vi "throw.vi"(8 "exception in":T1 {"code" format="%.0x"}, 11 "code":i32) -> (0 "exception":T1 {"code" format="%.0x"})   [LabVIEW 2013, in "exception.lvlib"]
uses:
  exception.lvlib
  exception.ctl
  context.ctl
  const exceptioncausename.vi
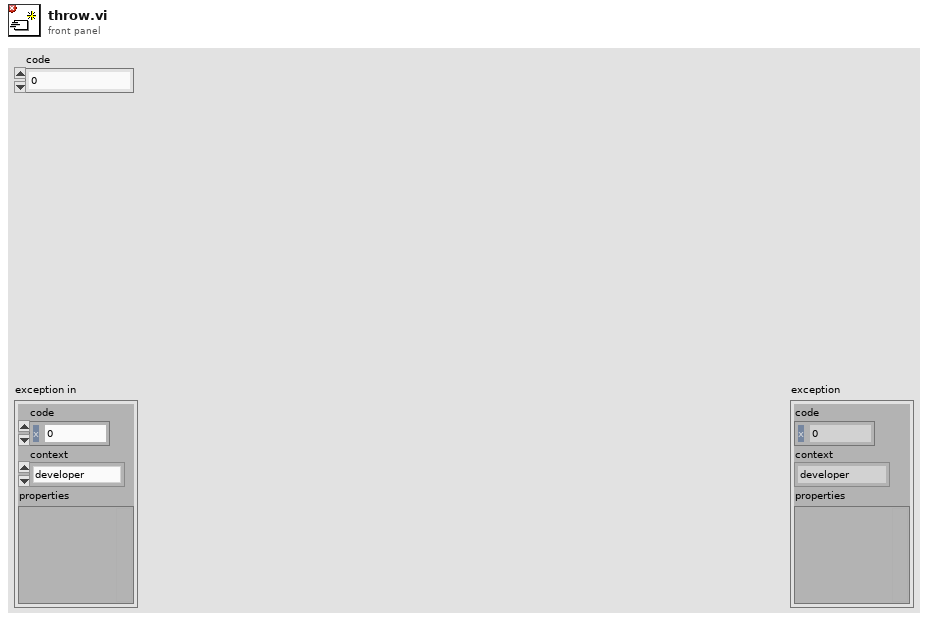
[diagram p1: front panel]
types:
  T1 = typedef "exception.lvlib/exception.ctl" = cluster{"code":i32, "context":T2, "properties":variant}
  T2 = typedef "exception.lvlib/context.ctl" = enum16{"developer", "user interface", "standard", "limited", "deterministic"}
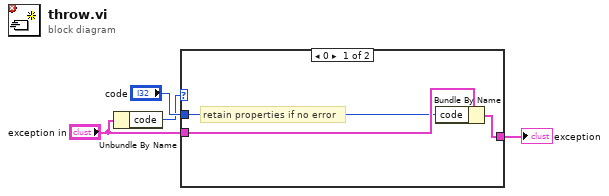
[diagram p0: block diagram]
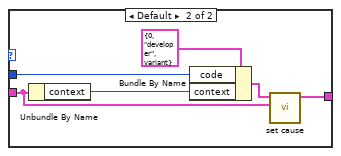
[diagram p2: hidden frame]
diagram:
  n1 = Unbundle By Name("exception in") -> ("code"=w1:i32)
  n2 = case shown="0" w1 {
    tunnel: [w6 w12] -> w4
    tunnel: "code" -> [w5 w10]
    tunnel: "exception in" -> [w7 w9]
    frame 0 {
      # "retain properties if no error"
      n3 = Bundle By Name(cluster=w7, "code"=w5) -> (w6:T1)
    }
    frame Default {
      n4 = Unbundle By Name(w9) -> ("context"=w8:T2)
      n5 = Bundle By Name(cluster=T1 {"code"=0, "context"=enum."developer", "properties"=variant} ("exception"), "code"=w10, "context"=w8) -> (w11:T1)
      n6 = call "set cause.vi"("cause"=w9, "exception in"=w11) -> ("exception out"=w12:T1)  [unwired: 9 in]
    }
  }
  "exception" <- w4
